vi "Show Search Results.vi"(8 "error in (no error)":errorcluster, 10 "Search":refnum<class "Search.lvclass">, 11 "BetterSearch in":refnum<class "BetterSearch.lvclass">) -> (0 "error out":errorcluster, 3 "BetterSearch out":refnum<class "BetterSearch.lvclass">)   [LabVIEW 2016, in "Better Search.lvlib" / "BetterSearch.lvclass"]
uses:
  BetterSearch.lvclass
  Search/Search.lvclass
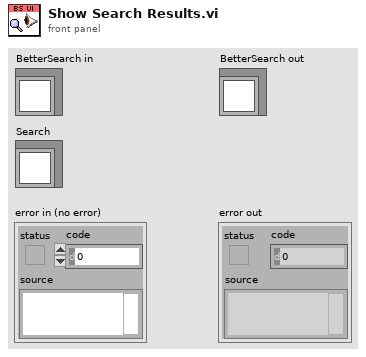
[diagram p1: front panel]
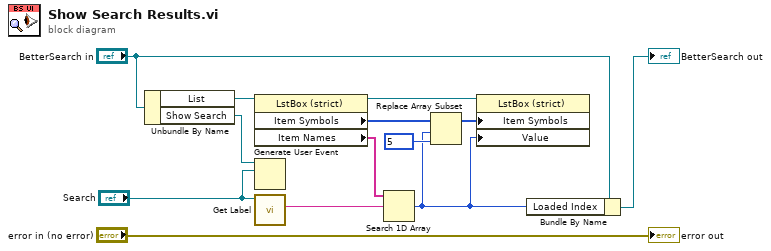
[diagram p0: block diagram]
diagram:
  n1 = Unbundle By Name("BetterSearch in") -> ("List"=w9:refnum<vi>, "Show Search"=w11:refnum<user-event>)
  n2 = property class="LstBox (strict)"(reference=w9) -> (reference out=w6:refnum<vi>, "Item Symbols"=w5:i32[], "Item Names"=w8:string[])  [unwired: 1 in, 1 out]
  n3 = Generate User Event(user event=w11, event data cluster="Search") -> ()  [unwired: 2 in, 2 out]
  n4 = call "Get Label.vi"("Search in"="Search") -> ("Label"=w7:string)  [unwired: 8 in, 2 out]
  n5 = Search 1D Array(1D array=w8, element=w7) -> (index of element=w1:i32)  [unwired: 1 in]
  n6 = Replace Array Subset(array=w5, new element=5, index=w1) -> (w4:i32[])
  n7 = property class="LstBox (strict)"(reference=w6, "Item Symbols"=w4, "Value"=w1) -> ()  [unwired: 1 in, 2 out]
  n8 = Bundle By Name(cluster="BetterSearch in", "Loaded Index"=w1) -> (→"BetterSearch out":refnum<class "BetterSearch.lvclass">)
  "error out" <- "error in (no error)"
